vi "fgv_AO_q.vi"(7 "cmd":T2, 8 "error in":errorcluster, 11 "data":T1) -> (0 "error out":errorcluster, 3 "queue out":refnum<queue>)   [LabVIEW 2019]
uses:
  _ctrl/create-rw-close.ctl
  AO_q-data.ctl
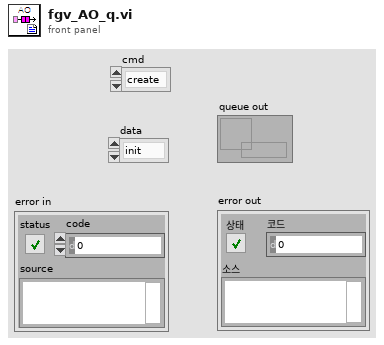
[diagram p1: front panel]
types:
  T1 = typedef "AO_q-data.ctl" = enum16{"init", "AO start"}
  T2 = typedef "create-rw-close.ctl" = enum16{"create", "write", "read", "delete", "close"}
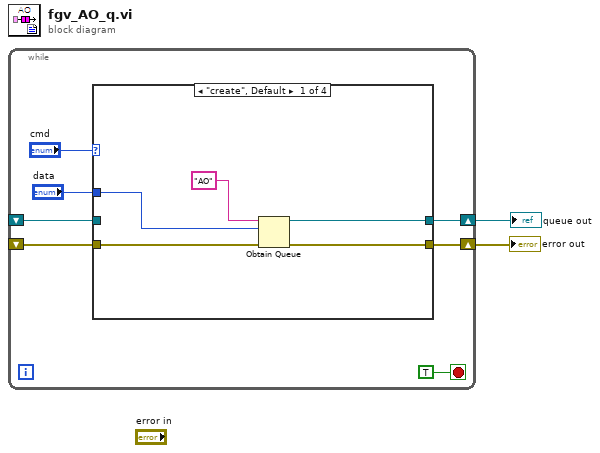
[diagram p0: block diagram]
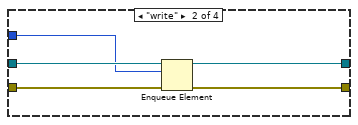
[diagram p2: hidden frame]
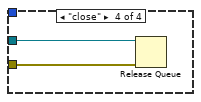
[diagram p4: hidden frame]
diagram:
  n1 = while {
    shift-right: [w6] -> w1
    shift-left: _ -> [w4]
    shift-right: [w5] -> w2
    shift-left: _ -> [w7]
    stop <- TRUE stop-if-true
    n2 = case shown="\"create\", Default" "cmd" {
      tunnel: w7 -> [w14 w18 w20 w23]
      tunnel: [w13 w17 w21 _] -> w6
      tunnel: [w12 w16 w20 _] -> w5
      tunnel: "data" -> [w10 w15 _ _]
      tunnel: w4 -> [_ w19 w21 w22]
      frame "create", Default {
        n3 = Obtain Queue(name (unnamed)="AO" ("이름(이름없음)"), element data type=w10, error in (no error)=w14) -> (queue out=w13:refnum<queue>, error out=w12:errorcluster)  [unwired: 2 in, 1 out]
      }
      frame "write" {
        n4 = Enqueue Element(queue=w19, element=w15, error in (no error)=w18) -> (queue out=w17:refnum<queue>, error out=w16:errorcluster)  [unwired: 1 in, 1 out]
      }
      frame "read" {
      }
      frame "close" {
        n5 = Release Queue(queue=w22, error in (no error)=w23) -> ()  [unwired: 1 in, 3 out]
      }
    }
  }
  "error out" <- w2
  "queue out" <- w1
